vi "Send Reply Msg DataSocket AE.vi"(6 "Timeout":i32, 7 "Message Priority (Normal)":T1=enum."Normal", 8 "error in":errorcluster, 9 "DataSocket Reply URL":string, 10 "Input":variant, 11 "Message Enqueuer":refnum<class "Message Enqueuer.lvclass">) -> (0 "error out":errorcluster, 1 "Timeout?":bool, 2 "Reply":variant, 3 "Message Enqueuer out":refnum<class "Message Enqueuer.lvclass">)   [LabVIEW 2023, in "Target Reply Time Test Actor.lvlib" / "Reply Msg DataSocket AE Msg.lvclass"]
doc: "This VI sends the message to an actor."
uses:
  Reply Msg DataSocket AE Msg.lvclass
  Reply Msg DataSocket AE Msg.lvclass/Reply Msg DataSocket AE Msg.ctl
  Reply Msg Host AE/Reply Msg DataSocket Connections Managed.lvclass
  <vilib>/ActorFramework/Message Enqueuer/Message Enqueuer.lvclass
  <vilib>/ActorFramework/Message Enqueuer/Message Priority.ctl
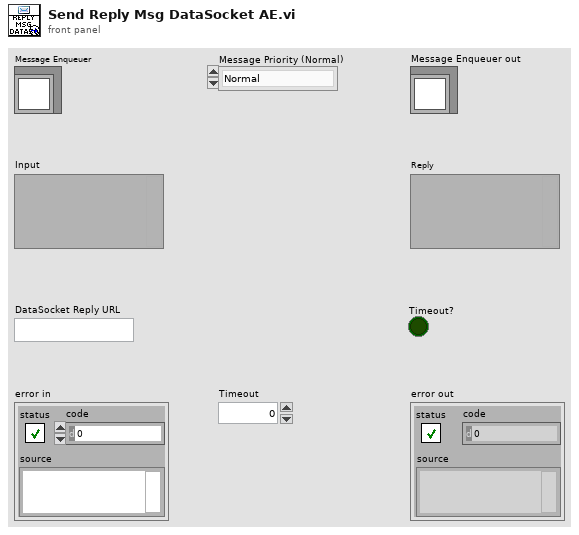
[diagram p1: front panel]
types:
  T1 = typedef "Actor Framework.lvlib/Message Enqueuer.lvclass/Message Priority.ctl" = enum16{"Low", "Normal", "High"}
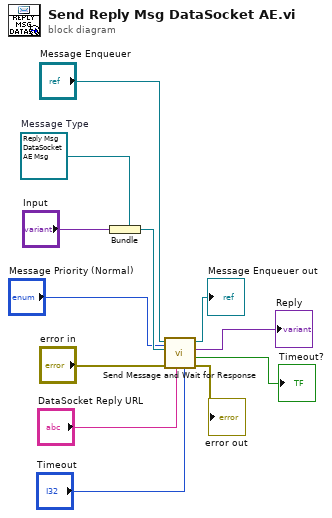
[diagram p0: block diagram]
diagram:
  w9 = refnum<class "Reply Msg DataSocket AE Msg.lvclass"> refnum  # Message Type
  n1 = Bundle(cluster=w9, "Input") -> (w8:refnum<class "Reply Msg DataSocket AE Msg.lvclass">)
  n2 = call "Send Message and Wait for Response.vi"("Timeout"="Timeout", "DataSocket Reply URL"="DataSocket Reply URL", "Message Priority (Normal)"="Message Priority (Normal)", "error in"="error in", "Original Message"=w8, "Message Enqueuer in"="Message Enqueuer") -> ("error out"=→"error out":errorcluster, "Timeout?"=→"Timeout?":bool, "Reply"=→"Reply":variant, "Message Enqueuer out"=→"Message Enqueuer out":refnum<class "Message Enqueuer.lvclass">)  [unwired: 2 in]
